vi "myRIO_BRig Hold Edge.vi"(0 "Trigger":bool, 1 "Reset?":bool) -> (2 "Signal?":bool)   [LabVIEW 2014]
panel:
  # "Signal? changes to true when a rising edge is detected on the Trigger input. The output is maintained at true unless the Reset? line is held high."
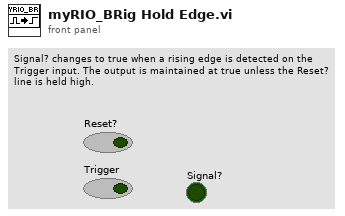
[diagram p1: front panel]
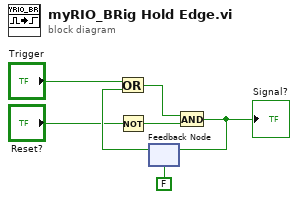
[diagram p0: block diagram]
diagram:
  n1 = Not(x="Reset?") -> (.not. x?=w3:bool)
  n2 = feedback #1(FALSE) -> (w7:bool)
  n3 = Or(x="Trigger", y=w7) -> (x .or. y?=w5:bool)
  n4 = And(x=w5, y=w3) -> (x .and. y?=w4:bool)
  "Signal?" <- w4
  n5 = feedback-in #1(w4) -> ()
